vi "Collect.vi"(1 "SpinupTrigger":bool, 2 "Firing Data":T2={"error"={"status"=FALSE, "code"=0, "source"=""}, "AngleMotorRefnum"={"DeviceStatus"={"status"=FALSE, "code"=0, "source"=""}, "Type"=enum."PWM", "PWM"={"PWM Channel"=enum."PWM 1", "DeadBand"={"Name"="", "maxPositivePwm"=0, "minPositivePwm"=0, "centerPwm"=0, "maxNegativePwm"=0, "minNegativePwm"=0, "angularRange"=0}}, "CAN"={"Device Number"=0, "Control Mode"=enum."Percent VBus", "Semaphore"=refnum, "Max Vout"=12.0, "TalonSRX Control Mode"=enum."Percent VBus"}, "Invert"=FALSE}, "LeftWheelRefnum"={"DeviceStatus"={"status"=FALSE, "code"=0, "source"=""}, "Type"=enum."PWM", "PWM"={"PWM Channel"=enum."Invalid", "DeadBand"={"Name"="", "maxPositivePwm"=0, "minPositivePwm"=0, "centerPwm"=0, "maxNegativePwm"=0, "minNegativePwm"=0, "angularRange"=0}}, "CAN"={"Device Number"=0, "Control Mode"=enum."Percent VBus", "Semaphore"=refnum, "Max Vout"=12.0, "TalonSRX Control Mode"=enum."Percent VBus"}, "Invert"=FALSE}, "RightWheelRefnum"={"DeviceStatus"={"status"=FALSE, "code"=0, "source"=""}, "Type"=enum."PWM", "PWM"={"PWM Channel"=enum."Invalid", "DeadBand"={"Name"="", "maxPositivePwm"=0, "minPositivePwm"=0, "centerPwm"=0, "maxNegativePwm"=0, "minNegativePwm"=0, "angularRange"=0}}, "CAN"={"Device Number"=0, "Control Mode"=enum."Percent VBus", "Semaphore"=refnum, "Max Vout"=12.0, "TalonSRX Control Mode"=enum."Percent VBus"}, "Invert"=FALSE}, "PushSolenoidRefnum"={"DevStatus"={"status"=FALSE, "code"=0, "source"=""}, "Pneumatics Control Module"=0, "Forward Solenoid Channel"=enum."Invalid", "Reverse Solenoid Channel"=enum."Invalid"}, "AngleMotorPosition(t)"=0.0, "LaunchSpeed(t/100ms)"=0.0, "CollectSpeed(t/100ms)"=0.0, "AngleThreshold"=0.0, "ShotDuration(10ms)"=0}, 3 "Manual Control":T1={"Joystick"=0.0, "LowerButton"=FALSE, "Aimbot?"=TRUE}, 4 "CollectionTrigger":bool) -> (0 "Firing Data":T2={"error"={"status"=FALSE, "code"=0, "source"=""}, "AngleMotorRefnum"={"DeviceStatus"={"status"=FALSE, "code"=0, "source"=""}, "Type"=enum."PWM", "PWM"={"PWM Channel"=enum."PWM 1", "DeadBand"={"Name"="", "maxPositivePwm"=0, "minPositivePwm"=0, "centerPwm"=0, "maxNegativePwm"=0, "minNegativePwm"=0, "angularRange"=0}}, "CAN"={"Device Number"=0, "Control Mode"=enum."Percent VBus", "Semaphore"=refnum, "Max Vout"=12.0, "TalonSRX Control Mode"=enum."Percent VBus"}, "Invert"=FALSE}, "LeftWheelRefnum"={"DeviceStatus"={"status"=FALSE, "code"=0, "source"=""}, "Type"=enum."PWM", "PWM"={"PWM Channel"=enum."Invalid", "DeadBand"={"Name"="", "maxPositivePwm"=0, "minPositivePwm"=0, "centerPwm"=0, "maxNegativePwm"=0, "minNegativePwm"=0, "angularRange"=0}}, "CAN"={"Device Number"=0, "Control Mode"=enum."Percent VBus", "Semaphore"=refnum, "Max Vout"=12.0, "TalonSRX Control Mode"=enum."Percent VBus"}, "Invert"=FALSE}, "RightWheelRefnum"={"DeviceStatus"={"status"=FALSE, "code"=0, "source"=""}, "Type"=enum."PWM", "PWM"={"PWM Channel"=enum."Invalid", "DeadBand"={"Name"="", "maxPositivePwm"=0, "minPositivePwm"=0, "centerPwm"=0, "maxNegativePwm"=0, "minNegativePwm"=0, "angularRange"=0}}, "CAN"={"Device Number"=0, "Control Mode"=enum."Percent VBus", "Semaphore"=refnum, "Max Vout"=12.0, "TalonSRX Control Mode"=enum."Percent VBus"}, "Invert"=FALSE}, "PushSolenoidRefnum"={"DevStatus"={"status"=FALSE, "code"=0, "source"=""}, "Pneumatics Control Module"=0, "Forward Solenoid Channel"=enum."Invalid", "Reverse Solenoid Channel"=enum."Invalid"}, "AngleMotorPosition(t)"=0.0, "LaunchSpeed(t/100ms)"=0.0, "CollectSpeed(t/100ms)"=0.0, "AngleThreshold"=0.0, "ShotDuration(10ms)"=0})   [LabVIEW 2015]
doc: "Collects boulders or aims manually."
uses:
  Bundle.ctl
  <vilib>/Rock Robotics/WPI/MotorControl/WPI_MotorControlDeviceRef.ctl
  <vilib>/Rock Robotics/WPI/MotorControl/WPI_MotorControlType.ctl
  <vilib>/Rock Robotics/SystemInterfaces/DIO/FPGA_DIOPWMChannel.ctl
  <vilib>/Rock Robotics/WPI/PWM/WPI_PWMDeadband.ctl
  <vilib>/Rock Robotics/WPI/CAN/Jaguar/SubVIs/WPI_CANJaguar_ControlMode.ctl
  <vilib>/Rock Robotics/WPI/CAN/TalonSRX/WPI_CANTalonSRX_APIControlMode.ctl
  <vilib>/Rock Robotics/WPI/Solenoid/WPI_SolenoidDevRef.ctl
  <vilib>/Rock Robotics/WPI/Solenoid/WPI_SolenoidChannel.ctl
  <vilib>/Rock Robotics/WPI/Solenoid/WPI_SolenoidValue.ctl
  <vilib>/Rock Robotics/WPI/Solenoid/WPI_SolenoidSetEnum.vi
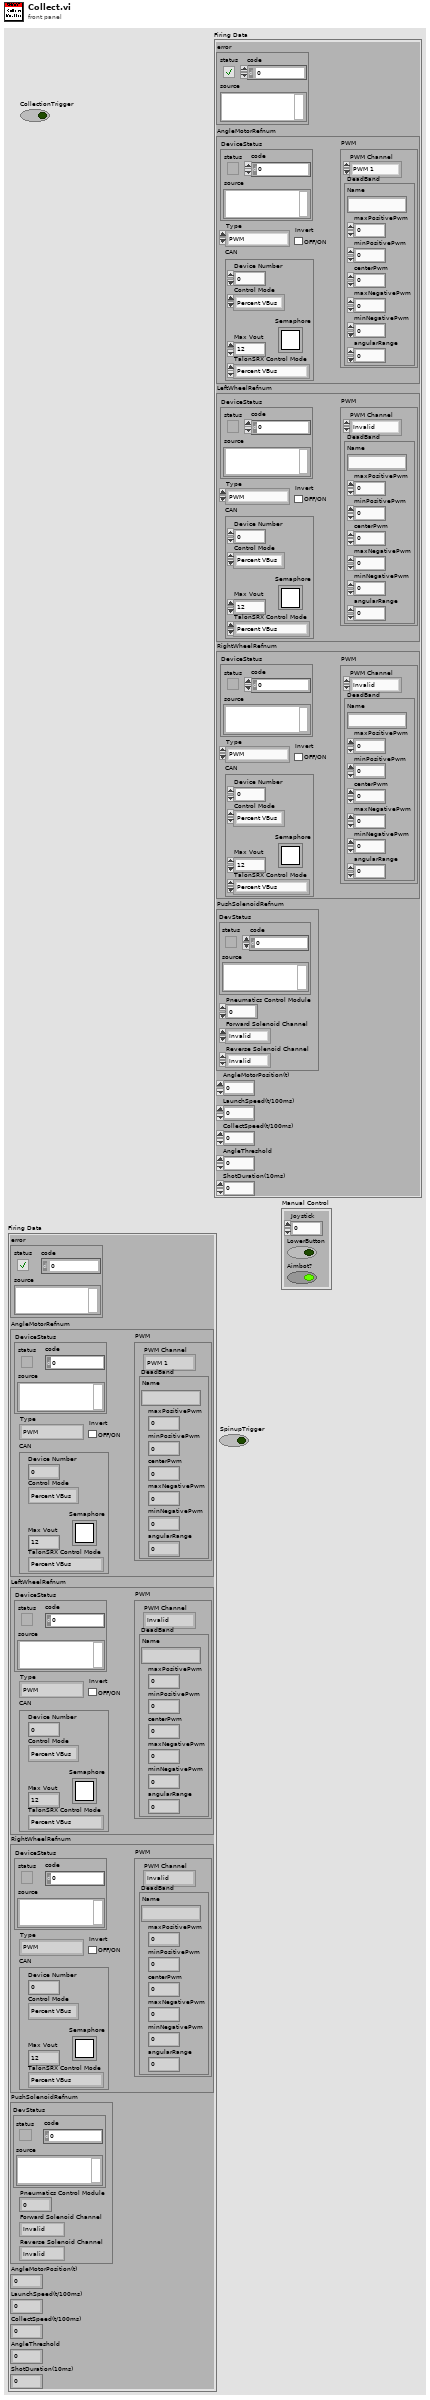
[diagram p1: front panel]
types:
  T1 = cluster{"Joystick":dbl, "LowerButton":bool, "Aimbot?":bool}
  T2 = typedef "Bundle.ctl" = cluster{"error":errorcluster, "AngleMotorRefnum":T3, "LeftWheelRefnum":T3, "RightWheelRefnum":T3, "PushSolenoidRefnum":T10, "AngleMotorPosition(t)":dbl, "LaunchSpeed(t/100ms)":dbl, "CollectSpeed(t/100ms)":dbl, "AngleThreshold":dbl, "ShotDuration(10ms)":i32}
  T3 = typedef "WPI_MotorControlDeviceRef.ctl" = cluster{"DeviceStatus":errorcluster, "Type":T4, "PWM":cluster{"PWM Channel":T5, "DeadBand":T6}, "CAN":cluster{"Device Number":u8, "Control Mode":T7, "Semaphore":T8, "Max Vout":dbl, "TalonSRX Control Mode":T9}, "Invert":bool}
  T4 = typedef "WPI_MotorControlType.ctl" = enum16{"PWM", "CAN", "CANTalonSRX"}
  T5 = typedef "FPGA_DIOPWMChannel.ctl" = enum8{"PWM 0", "PWM 1", "PWM 2", "PWM 3", "PWM 4", "PWM 5", "PWM 6", "PWM 7", "PWM 8", "PWM 9", "PWM MXP 0", "PWM MXP 1", "PWM MXP 2", "PWM MXP 3", "PWM MXP 4", "PWM MXP 5", "PWM MXP 6", "PWM MXP 7", "PWM MXP 8", "PWM MXP 9", "Invalid"}
  T6 = typedef "WPI_PWMDeadband.ctl" = cluster{"Name":string, "maxPositivePwm":i32, "minPositivePwm":i32, "centerPwm":i32, "maxNegativePwm":i32, "minNegativePwm":i32, "angularRange":u16}
  T7 = typedef "WPI_CANJaguar_ControlMode.ctl" = enum8{"Percent VBus", "Current", "Speed", "Position", "Voltage"}
  T8 = typedef "Semaphore RefNum" = refnum<k1>
  T9 = typedef "WPI_CANTalonSRX_APIControlMode.ctl" = enum8{"Percent VBus", "Speed", "Position", "Slave", "Unchanged / Invalid", "Voltage Compensation", "Current", "Motion Profile"}
  T10 = typedef "WPI_SolenoidDevRef.ctl" = cluster{"DevStatus":errorcluster, "Pneumatics Control Module":u8, "Forward Solenoid Channel":T11, "Reverse Solenoid Channel":T11}
  T11 = typedef "WPI_SolenoidChannel.ctl" = enum8{"Solenoid 0", "Solenoid 1", "Solenoid 2", "Solenoid 3", "Solenoid 4", "Solenoid 5", "Solenoid 6", "Solenoid 7", "Invalid"}
  T12 = typedef "WPI_SolenoidValue.ctl" = enum16{"Off", "On", "Forward", "Reverse"}
  T13 = typedef "WPI_CANTalonSRX_GlobalStatus.ctl" = cluster{"Applied Throttle":dbl, "Module Enabled":bool, "CAN Error":errorcluster, "Closed Loop Error":dbl, "Forward Limit Switch Closed":bool, "Reverse Limit Switch Closed":bool, "Sensor Position":dbl, "Sensor Velocity":dbl, "Current":dbl, "Sticky Fault - Over Temp":bool, "Sticky Fault - Under Voltage":bool, "Sticky Fault - Forward Limit":bool, "Sticky Fault - Reverse Limit":bool, "Sticky Fault - Forward Soft Limit":bool, "Sticky Fault - Reverse Soft Limit":bool, "Brake is Enabled":bool, "Encoder Position":dbl, "Encoder Velocity":dbl, "Encoder Index Count":dbl, "Encoder A Pin State":bool, "Encoder B Pin State":bool, "Encoder Index Pin State":bool, "Analog In":dbl, "Analog In Velocity":dbl, "Temperature (C)":dbl, "Battery Voltage":dbl, "Control 5 Is Supported":bool, "Current Profile Slot Select":dbl, "Pos Div 8":bool, "Vel Div 4":bool, "Pulse Width Position":i32, "Pulse Width Velocity":i32, "Pulse Width Rise To Rise (us)":i32, "Pulse Width Rise To Fall (us)":i32, "Mot Prof Active Is Under Run":bool, "Mot Prof Active Has Under Run":bool, "Mot Prof Active Is Last":bool, "Mot Prof Active Velocity Only":bool, "Mot Prof Active Is Valid":bool, "Mot Prof Buffer Is Full":bool, "Mot Prof Active Profile Slot Select":i32, "Mot Prof NextID":i32, "Mot Prof Count":i32, "Mot Prof Active Velocity":dbl, "Mot Prof Active Position":dbl, "Mot Prof Output Enable":i32}
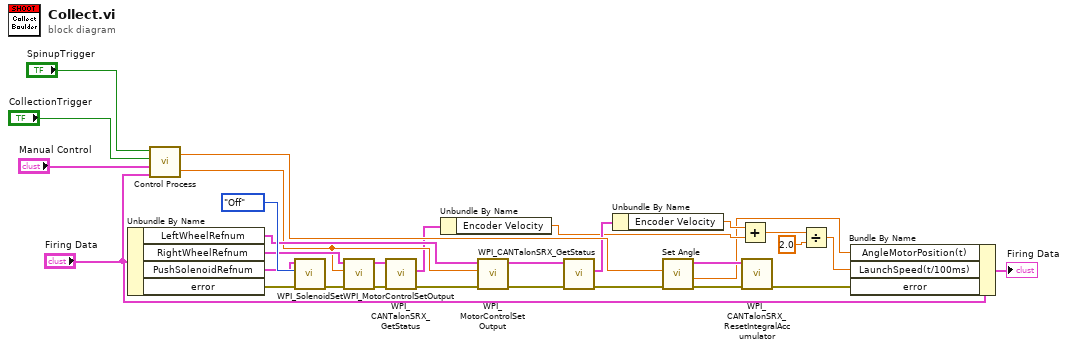
[diagram p0: block diagram]
diagram:
  n1 = Unbundle By Name("Firing Data") -> ("LeftWheelRefnum"=w22:T3, "RightWheelRefnum"=w21:T3, "PushSolenoidRefnum"=w25:T10, "error"=w26:errorcluster)
  n2 = call "Control Process.vi"("Firing Data"="Firing Data", "Manual Control"="Manual Control", "CollectionTrigger"="CollectionTrigger", "SpinupTrigger"="SpinupTrigger") -> ("Speed"=w19:dbl, "Angle"=w20:dbl)
  n3 = call-poly <vilib>:"WPI_SolenoidSet.vi"("error in (no error)"=w26, "Value"=WPI_SolenoidValue."Off", "SolenoidDevRef"=w25) -> ("error out"=w23:errorcluster)  [unwired: 7 in, 1 out]
  n4 = call <vilib>:"WPI_MotorControlSetOutput.vi"("error in (no error)"=w23, "Output"=w19, "MotorControlDevRef"=w21) -> ("error out"=w7:errorcluster, "MotorControlDevRef"=w9:T3)  [unwired: 6 in, 1 out]
  n5 = call <vilib>:"WPI_CANTalonSRX_GetStatus.vi"("error in (no error)"=w7, "CAN Talon SRX Ref"=w9) -> ("error out"=w6:errorcluster, "Talon SRX Status"=w13:T13)  [unwired: 7 in, 1 out]
  n6 = Unbundle By Name(w13) -> ("Encoder Velocity"=w11:dbl)
  n7 = call <vilib>:"WPI_MotorControlSetOutput.vi"("error in (no error)"=w6, "Output"=w19, "MotorControlDevRef"=w22) -> ("error out"=w4:errorcluster, "MotorControlDevRef"=w10:T3)  [unwired: 6 in, 1 out]
  n8 = call <vilib>:"WPI_CANTalonSRX_GetStatus.vi"("error in (no error)"=w4, "CAN Talon SRX Ref"=w10) -> ("error out"=w5:errorcluster, "Talon SRX Status"=w14:T13)  [unwired: 7 in, 1 out]
  n9 = Unbundle By Name(w14) -> ("Encoder Velocity"=w12:dbl)
  n10 = call "Set Angle.vi"("error in (no error)"=w5, "Angle(degrees)"=w20) -> ("error out"=w29:errorcluster, "Pot Position"=w3:dbl, "Angle Refnum"=w28:T3)  [unwired: 6 in, 1 out]
  n11 = Add(x=w12, y=w11) -> (x+y=w15:dbl)
  n12 = call <vilib>:"WPI_CANTalonSRX_ResetIntegralAccumulator.vi"("error in (no error)"=w29, "CAN Talon SRX Ref"=w28) -> ("error out"=w2:errorcluster)  [unwired: 8 in, 1 out]
  n13 = Divide(x=w15, y=2.0) -> (x/y=w8:dbl)
  n14 = Bundle By Name(cluster="Firing Data", "AngleMotorPosition(t)"=w3, "LaunchSpeed(t/100ms)"=w8, "error"=w2) -> (→"Firing Data":T2)
